vi "Apply Weight Precheck.vi"(8 "error in (no error)":errorcluster, 9 "Slot Number":i32, 10 "Chuck Number":i32, 11 "GrabberTool Class in":refnum<class "GrabberTool Class.lvclass">) -> (0 "error out":errorcluster, 3 "GrabberTool Class out":refnum<class "GrabberTool Class.lvclass">)   [LabVIEW 2011, in "GrabberTool Class.lvclass"]
uses:
  GrabberTool Class.lvclass
  WorkTable Class/WorkTable Class.lvclass
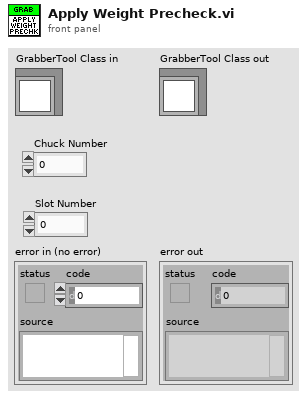
[diagram p1: front panel]
types:
  T1 = typedef "Worktable_Module Slot.ctl" = cluster{"Slot State":enum16{"Empty", "Unglued", "Stamped", "PartOnTop", "Weighted", "Unpotted", "Potted"}, "BBM Type":enum16{"None", "BBM", "GlassSlide"}, "HDI Type":enum16{"None", "HDI", "Polyimide"}, "Vacuum Channel":u8, "Location/Orientation BBM":T2, "Location/Orientation HDI":T2, "S/N":string}
  T2 = typedef "Position_Orientation.ctl" = cluster{"Center":refnum<class "Vec3d Class.lvclass">, "Orientation":refnum<class "Orient3d Class.lvclass">}
  T3 = enum16{"Empty", "Unglued", "Stamped", "PartOnTop", "Weighted", "Unpotted", "Potted"}
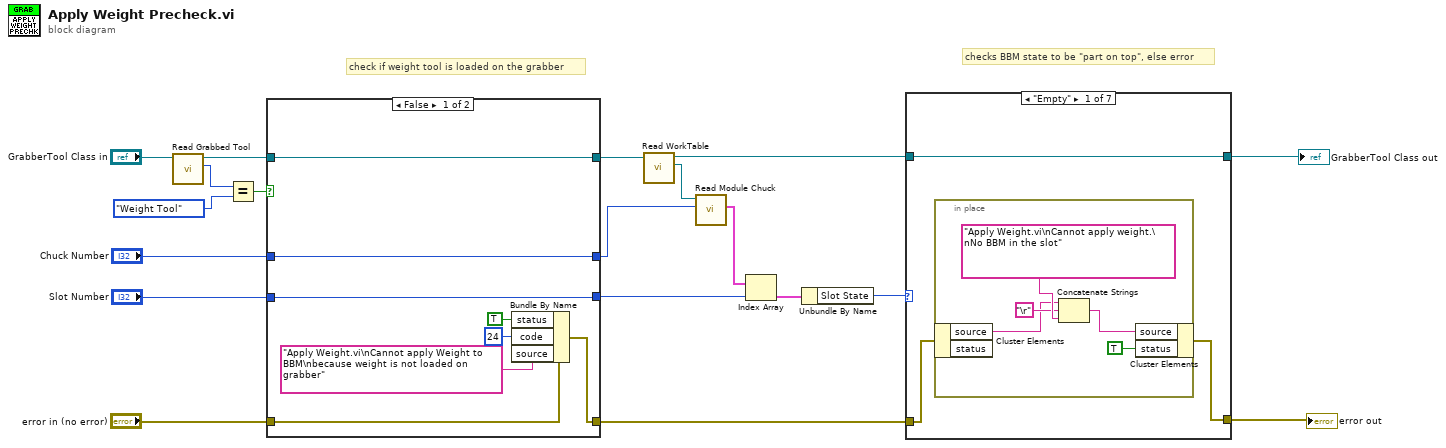
[diagram p0: block diagram]
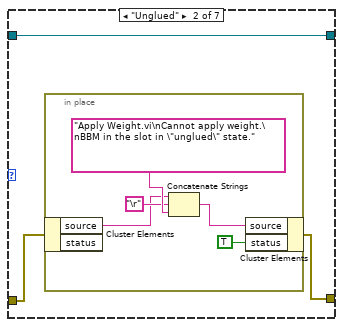
[diagram p2: hidden frame]
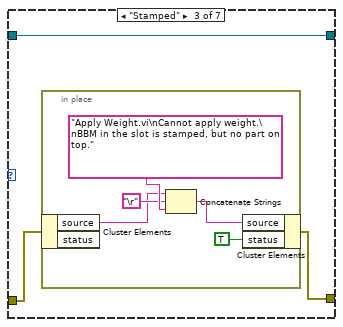
[diagram p3: hidden frame]
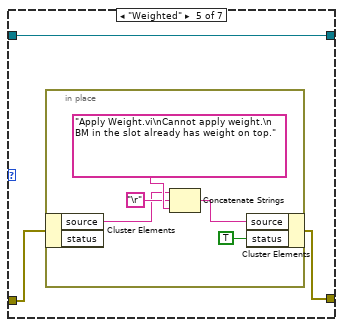
[diagram p5: hidden frame]
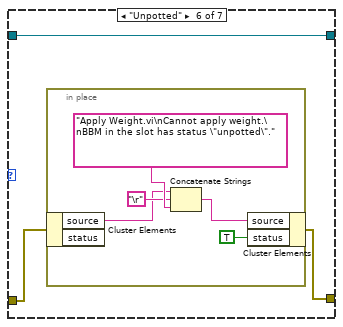
[diagram p6: hidden frame]
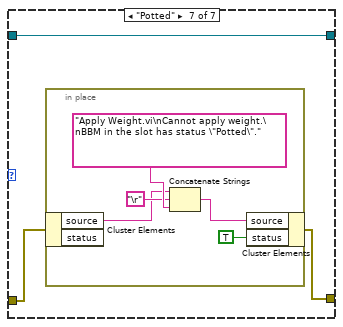
[diagram p7: hidden frame]
diagram:
  # "checks BBM state to be \"part on top\", else error"
  # "check if weight tool is loaded on the grabber"
  n1 = call "Read Grabbed Tool.vi"("GrabberTool Class in"="GrabberTool Class in") -> ("Grabbed Tool"=w18:enum16{"Weight Tool", "Stamp Tool", "Nothing"}, "GrabberTool Class out"=w15:refnum<class "GrabberTool Class.lvclass">)  [unwired: 8 in, 1 out]
  n2 = Equal?(x=w18, y=enum16{"Weight Tool", "Stamp Tool", "Nothing"}."Weight Tool" ("Grabbed Tool")) -> (x = y?=w16:bool)
  n3 = case shown="False" w16 {
    tunnel: [w22 w30] -> w3
    tunnel: [w27 w31] -> w8
    tunnel: w15 -> [w27 w31]
    tunnel: "error in (no error)" -> [w23 w30]
    tunnel: "Chuck Number" -> [w21 w29]
    tunnel: [w21 w29] -> w7
    tunnel: [w20 w28] -> w6
    tunnel: "Slot Number" -> [w20 w28]
    frame False {
      n4 = Bundle By Name(cluster=w23, "status"=TRUE, "code"=24, "source"="Apply Weight.vi\nCannot apply Weight to BBM\nbecause weight is not loaded on grabber") -> (w22:errorcluster)
    }
    frame True {
    }
  }
  n5 = call-dynamic "Read WorkTable.vi"("Gantry Class in"=w8) -> ("WorkTable Class.lvclass"=w11:refnum<class "WorkTable Class.lvclass">, "Gantry Class out"=w4:refnum<class "GrabberTool Class.lvclass">)  [unwired: 8 in, 1 out]
  n6 = call-dynamic "Read Module Chuck.vi"("index"=w7, "WorkTable in"=w11) -> ("Module Slots"=w10:T1[])  [unwired: 7 in, 2 out]
  n7 = Index Array(array=w10, index=w6) -> (element=w9:T1)
  n8 = Unbundle By Name(w9) -> ("Slot State"=w5:T3)
  n9 = case shown="\"Empty\"" w5 {
    tunnel: w4 -> [w32 w40 w48 w57 w58 w66 w74]
    tunnel: w3 -> [w34 w42 w50 w56 w60 w68 w76]
    tunnel: [w33 w41 w49 w56 w59 w67 w75] -> w2
    tunnel: [w32 w40 w48 w57 w58 w66 w74] -> w1
    frame "Empty" {
      n10 = in-place {
        n11 = in-place-cluster #1(w34) -> ("source"=w36:string)  [unwired: 1 out]
        n12 = Concatenate Strings(w36, "\r", "Apply Weight.vi\nCannot apply weight.\nNo BBM in the slot" ("string")) -> (w37:string)
        n13 = in-place-cluster #1("source"=w37, "status"=TRUE) -> (w33:errorcluster)
      }
    }
    frame "Unglued" {
      n14 = in-place {
        n15 = in-place-cluster #2(w42) -> ("source"=w44:string)  [unwired: 1 out]
        n16 = Concatenate Strings(w44, "\r", "Apply Weight.vi\nCannot apply weight.\nBBM in the slot in \"unglued\" state." ("string")) -> (w45:string)
        n17 = in-place-cluster #2("source"=w45, "status"=TRUE) -> (w41:errorcluster)
      }
    }
    frame "Stamped" {
      n18 = in-place {
        n19 = in-place-cluster #3(w50) -> ("source"=w52:string)  [unwired: 1 out]
        n20 = Concatenate Strings(w52, "\r", "Apply Weight.vi\nCannot apply weight.\nBBM in the slot is stamped, but no part on top." ("string")) -> (w53:string)
        n21 = in-place-cluster #3("source"=w53, "status"=TRUE) -> (w49:errorcluster)
      }
    }
    frame "PartOnTop" {
    }
    frame "Weighted" {
      n22 = in-place {
        n23 = in-place-cluster #4(w60) -> ("source"=w62:string)  [unwired: 1 out]
        n24 = Concatenate Strings(w62, "\r", "Apply Weight.vi\nCannot apply weight.\n BM in the slot already has weight on top." ("string")) -> (w63:string)
        n25 = in-place-cluster #4("source"=w63, "status"=TRUE) -> (w59:errorcluster)
      }
    }
    frame "Unpotted" {
      n26 = in-place {
        n27 = in-place-cluster #5(w68) -> ("source"=w70:string)  [unwired: 1 out]
        n28 = Concatenate Strings(w70, "\r", "Apply Weight.vi\nCannot apply weight.\nBBM in the slot has status \"unpotted\"." ("string")) -> (w71:string)
        n29 = in-place-cluster #5("source"=w71, "status"=TRUE) -> (w67:errorcluster)
      }
    }
    frame "Potted" {
      n30 = in-place {
        n31 = in-place-cluster #6(w76) -> ("source"=w78:string)  [unwired: 1 out]
        n32 = Concatenate Strings(w78, "\r", "Apply Weight.vi\nCannot apply weight.\nBBM in the slot has status \"Potted\"." ("string")) -> (w79:string)
        n33 = in-place-cluster #6("source"=w79, "status"=TRUE) -> (w75:errorcluster)
      }
    }
  }
  "error out" <- w2
  "GrabberTool Class out" <- w1
